vi "distancesEdges(SubVI).vi"(8 "error in (no error)":errorcluster, 9 "Edge Information":T2[](array[typedef]) {"Distance (Real-World)" format="%.2f"; "Location (Real-World)"."Y" format="%.2g"; "Location (Real-World)"."X" format="%.2f"; "Noise" format="%.2f"; "Location (Pixel)"."Y" format="%.2g"; "Location (Pixel)"."X" format="%.2f"; "Strength" format="%.2f"; "Distance (Pixel)" format="%.2f"}, 11 "Image In":T1) -> (0 "error out":errorcluster)   [LabVIEW 2020]
uses:
  <vilib>/vision/Measure.llb/Edge New.ctl
  <vilib>/vision/Image Controls.llb/IMAQ Image.ctl
  <vilib>/vision/NI_Vision_Development_Module.lvlib
panel:
  out "String":string
  in  "Real word":bool
  out "Image 2":T1(plugin-control)
  in  "index":i32
  in  "index 2":i32
  in  "stop":bool
  # "Pixel"
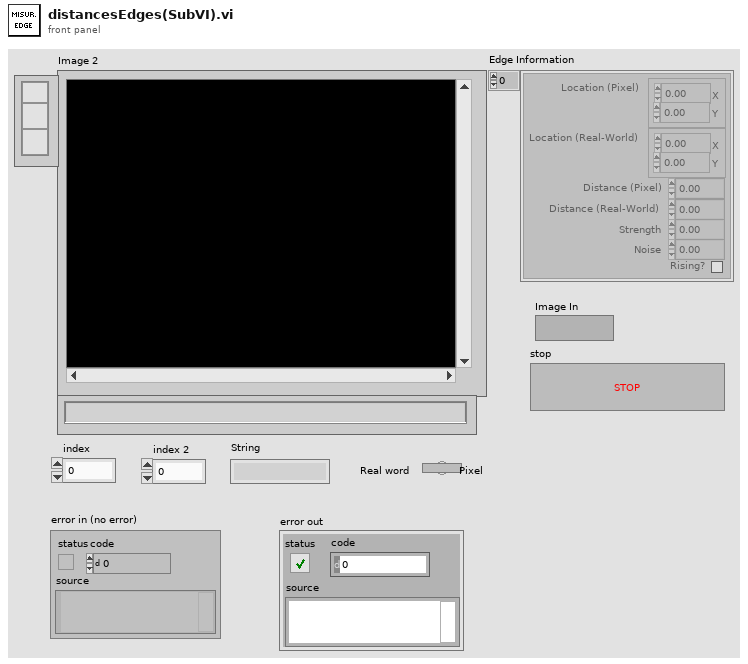
[diagram p1: front panel]
types:
  T1 = typedef "IMAQ Image.ctl" = refnum<image>
  T2 = typedef "Edge New.ctl" = cluster{"Location (Pixel)":cluster{"X":sgl, "Y":sgl}, "Location (Real-World)":cluster{"X":sgl, "Y":sgl}, "Distance (Pixel)":dbl, "Distance (Real-World)":dbl, "Strength":dbl, "Noise":dbl, "Rising?":bool}
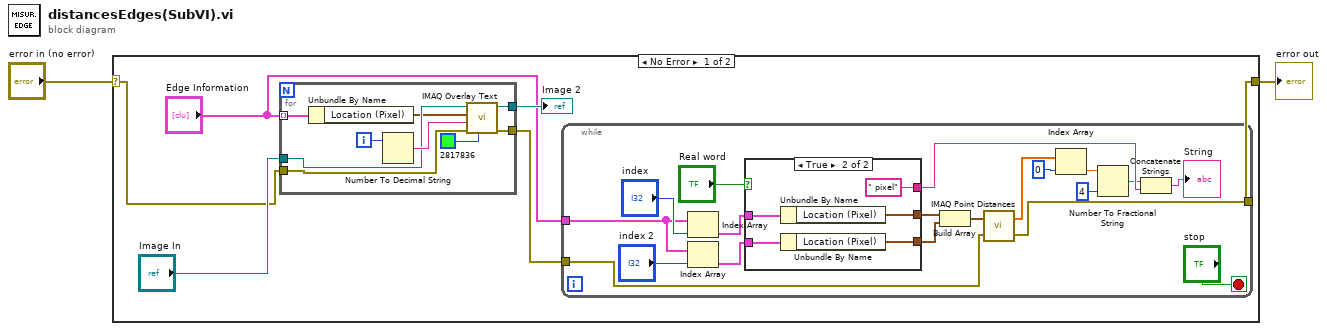
[diagram p0: block diagram]
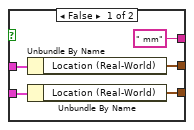
[diagram p2: hidden frame]
diagram:
  n1 = case shown="No Error" "error in (no error)" {
    selector: "error in (no error)" -> [w5 w47]
    tunnel: [w3 w47] -> w1
    frame No Error {
      n2 = for {
        tunnel: "Image In" -> [w15]
        tunnel: [w12] -> w8
        tunnel: "Edge Information" -> [w11] mode=indexing
        tunnel: w5 -> [w10]
        tunnel: [w9] -> w4
        i -> [w17]
        n3 = Unbundle By Name(w11) -> ("Location (Pixel)"=w14:cluster{"X":sgl, "Y":sgl})
        n4 = Number To Decimal String(number=w17) -> (decimal integer string=w16:string)  [unwired: 1 in]
        n5 = call "IMAQ Overlay Text"("Text Color (black)"=u32 2817836, "error in (no error)"=w10, "String"=w16, "Origin"=w14, "Image"=w15) -> ("error out"=w9:errorcluster, "Image Out"=w12:T1)  [unwired: 5 in]
      }
      "Image 2" <- w8
      n6 = while {
        tunnel: "Edge Information" -> [w28]
        tunnel: w4 -> [w27]
        tunnel: [w26] -> w3
        stop <- "stop" stop-if-true
        n7 = Index Array(array=w28, index="index") -> (element=w33:T2)
        n8 = Index Array(array=w28, index="index 2") -> (element=w32:T2)
        n9 = case shown="True" "Real word" {
          tunnel: w33 -> [w41 w46]
          tunnel: w32 -> [w39 w45]
          tunnel: [w40 w44] -> w30
          tunnel: [w38 w43] -> w29
          tunnel: [" mm" " pixel"] -> w24
          frame False {
            n10 = Unbundle By Name(w41) -> ("Location (Real-World)"=w40:cluster{"X":sgl, "Y":sgl})
            n11 = Unbundle By Name(w39) -> ("Location (Real-World)"=w38:cluster{"X":sgl, "Y":sgl})
          }
          frame True {
            n12 = Unbundle By Name(w46) -> ("Location (Pixel)"=w44:cluster{"X":sgl, "Y":sgl})
            n13 = Unbundle By Name(w45) -> ("Location (Pixel)"=w43:cluster{"X":sgl, "Y":sgl})
          }
        }
        n14 = Build Array(w30, w29) -> (w31:cluster{"X":sgl, "Y":sgl}[])
        n15 = call "IMAQ Point Distances"("Points"=w31, "error in (no error)"=w27) -> ("Distances"=w23:sgl[], "error out"=w26:errorcluster)  [unwired: 3 in]
        n16 = Index Array(array=w23, index=0) -> (element=w20:sgl)
        n17 = Number To Fractional String(number=w20, precision (6)=i16 4) -> (F-format string=w19:string)  [unwired: 2 in]
        n18 = Concatenate Strings(w19, w24) -> (→"String":string)
      }
    }
    frame Error {
    }
  }
  "error out" <- w1
